vi "3.7-Reliable UPD Client Template.vi"() -> ()   [LabVIEW 2010]
uses:
  3.0-Global.vi
panel:
  out "My Global Variable":cluster{i32, bool}
  in  "error in":errorcluster={"status"=TRUE, "code"=0, "source"=""}
  out "error out":errorcluster
  in  "stop":bool
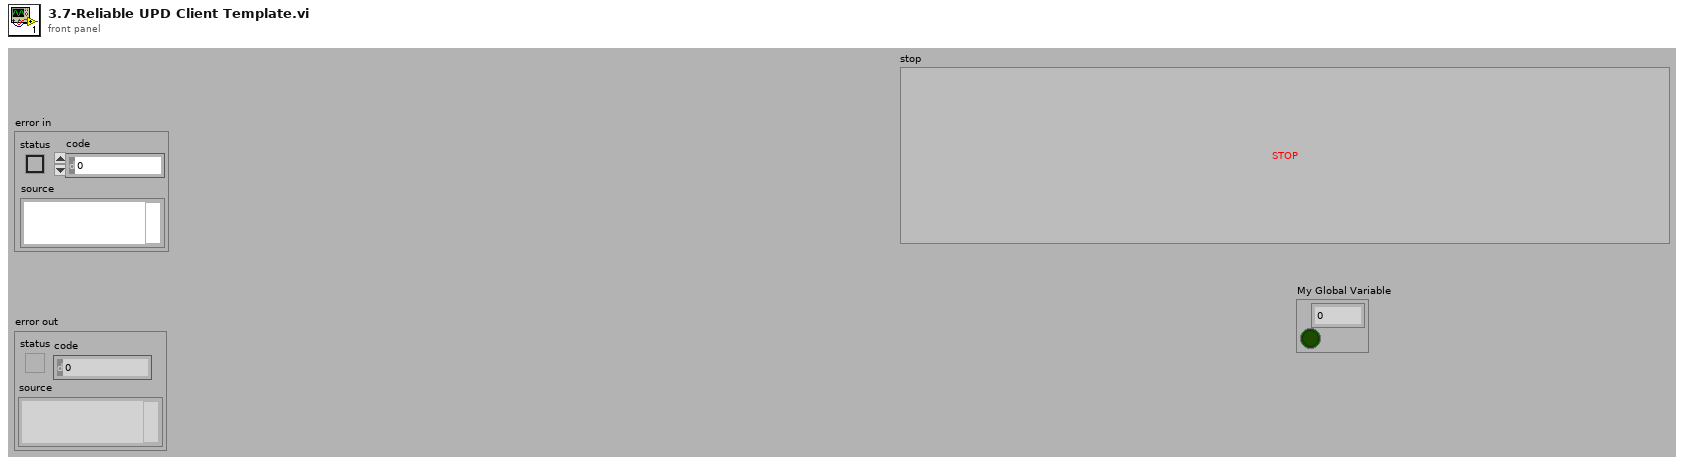
[diagram p1: front panel]
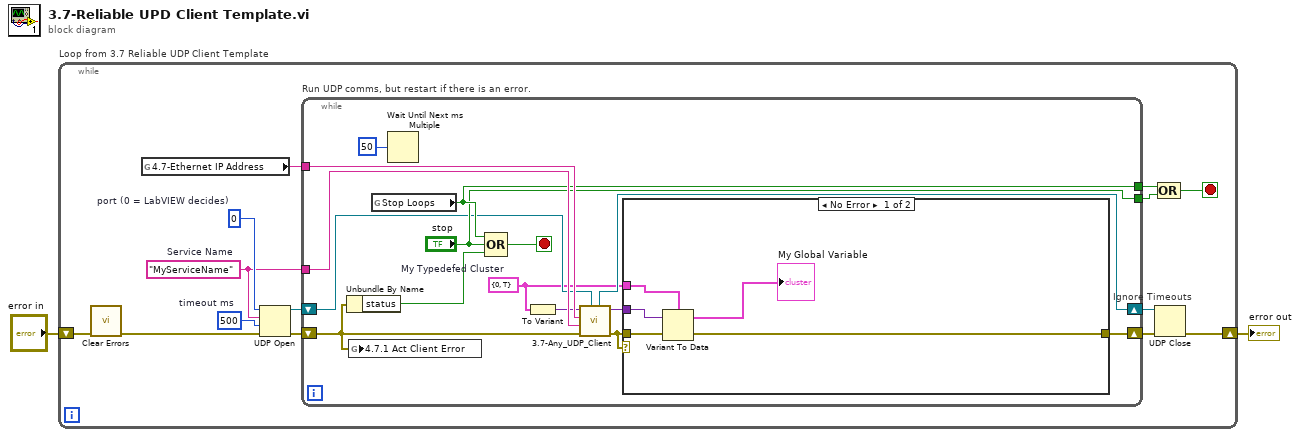
[diagram p0: block diagram]
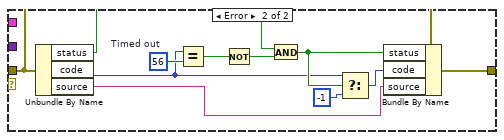
[diagram p2: hidden frame]
diagram:
  n1 = while "Loop from 3.7 Reliable UDP Client Template" {
    shift-right: [w9] -> w1
    shift-left: "error in" -> [w5]
    stop <- w14 stop-if-true
    w6 = 500  # timeout ms
    w8 = u16 0  # port (0 = LabVIEW decides)
    w7 = "MyServiceName"  # Service Name
    n2 = call <vilib>:"Clear Errors.vi"("error in (no error)"=w5) -> ("error out"=w4:errorcluster)  [unwired: 6 in]
    n3 = global read "3.0-Global.vi" "4.7-Ethernet IP Address"() -> (w3:string)
    n4 = UDP Open(8:w4, 9:w6, 10:w7, 11:w8) -> (port=w13:refnum<k16>, 0:w11:errorcluster)  [unwired: 1 in, 1 out]
    n5 = while "Run UDP comms, but restart if there is an error." {
      tunnel: w7 -> [w28]
      tunnel: w3 -> [w29]
      tunnel: [w25] -> w16
      tunnel: ["stop"] -> w15
      shift-right: [w21] -> w12
      shift-left: w13 -> [w22]
      shift-right: [w20] -> w10
      shift-left: w11 -> [w18]
      stop <- w31 stop-if-true
      w17 = cluster{i32, bool} {0, TRUE}  # My Typedefed Cluster
      n6 = Unbundle By Name(w18) -> ("status"=w23:bool)
      n7 = global write "3.0-Global.vi" "4.7.1 Act Client Error"(w18) -> ()
      n8 = global read "3.0-Global.vi" "Stop Loops"() -> (w25:bool)
      n9 = Wait Until Next ms Multiple(millisecond multiple=u32 50) -> ()  [unwired: 1 out]
      n10 = Compound Arithmetic op=OR(w25, "stop", w23) -> (w31:bool)
      n11 = To Variant(anything=w17) -> (Variant=w27:variant)
      n12 = call "3.7-Any_UDP_Client.vi"("Port In"=w22, "error In"=w18, "Service Name"=w28, "IP Address"=w29, "DataTypeIn"=w27) -> ("Error Out"=w19:errorcluster, "DataOut"=w26:variant, "Port out"=w21:refnum<k16>)  [unwired: 3 in, 1 out]
      n13 = case "Ignore Timeouts" shown="No Error" w19 {
        tunnel: w26 -> [w36 _]
        tunnel: w17 -> [w35 _]
        tunnel: w19 -> [w34 w47]
        tunnel: [w33 w46] -> w20
        frame No Error {
          n14 = Variant To Data(error in=w34, Variant=w36, type=w35) -> (error out=w33:errorcluster, data=→"My Global Variable":cluster{i32, bool})
        }
        frame Error {
          w45 = 56  # Timed out
          n15 = Unbundle By Name(w47) -> ("status"=w42:bool, "code"=w40:i32, "source"=w37:string)
          n16 = Equal?(x=w40, y=w45) -> (x = y?=w44:bool)
          n17 = Not(x=w44) -> (.not. x?=w43:bool)
          n18 = And(x=w42, y=w43) -> (x .and. y?=w41:bool)
          n19 = Select(t=w40, s=w41, f=-1) -> (s? t:f=w38:i32)
          n20 = Bundle By Name(cluster=w47, "status"=w41, "code"=w38, "source"=w37) -> (w46:errorcluster)
        }
      }
    }
    n21 = UDP Close(connection ID=w12, 8:w10) -> (error out=w9:errorcluster)  [unwired: 1 out]
    n22 = Compound Arithmetic op=OR(w16, w15) -> (w14:bool)
  }
  "error out" <- w1
